vi "SOUR_POW_CORR_COLL_ABOR.vi"(0 "VISA IN":refnum<visa-resource-name>, 1 "Port number":i32, 5 "error in":errorcluster, 7 "Channel":i32) -> (14 "VISA Out":refnum<visa-resource-name>, 19 "error out":errorcluster)   [LabVIEW 2018, in "PNA-X.lvlib"]
doc: "SOURce<cnum>:POWer<port>:CORRection:COLLect:ABORt \n1834\n\n(Write-only) Aborts a source power calibration sweep that is in progress. \nParameters \n<cnum> Any existing channel number. If unspecified, value is set to 1 \n<port> Port number to correct for source power. If unspecified, value is set to 1. \nExamples SOUR:POW:CORR:COLL:ABOR \nsource1:power2:correction:collect:abort \nQuery Syntax Not Applicable \nDefault Not Applicable"
uses:
  PNA-X.lvlib
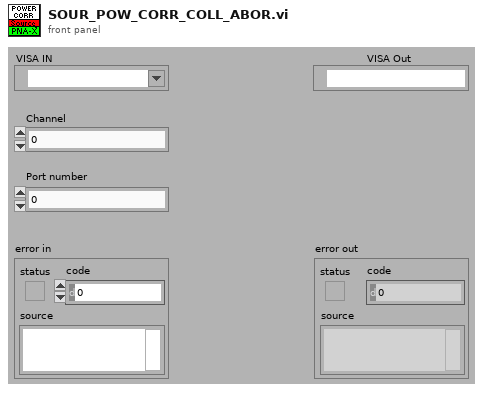
[diagram p1: front panel]
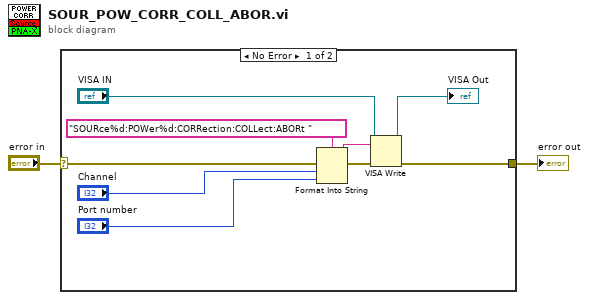
[diagram p0: block diagram]
diagram:
  n1 = case shown="No Error" "error in" {
    selector: "error in" -> [w11 w12]
    tunnel: [w6 w12] -> w1
    frame No Error {
      n2 = Format Into String(format string="SOURce%d:POWer%d:CORRection:COLLect:ABORt " ("Cmdline"), error in=w11, "Channel", "Port number") -> (resulting string=w9:string, error out=w10:errorcluster)  [unwired: 1 in]
      n3 = VISA Write(VISA resource name="VISA IN", write buffer=w9, error in (no error)=w10) -> (VISA resource name out=→"VISA Out":refnum<visa-resource-name>, error out=w6:errorcluster)  [unwired: 1 out]
    }
    frame Error {
    }
  }
  "error out" <- w1
